vi "Stop Shooter.vi"   [LabVIEW 2013]
uses:
  Shooter Manual Control.ctl
  Shooter Command.ctl
  Robot Global Data.vi
types:
  T1 = typedef "Shooter Manual Control.ctl" = cluster{"Command":T2, "Offset":dbl, "Trigger":bool, "Add":bool, "Release":bool, "Reset":bool, "Target Pressure":dbl, "Punch":bool, "AutoPunch":bool}
  T2 = typedef "Shooter Command.ctl" = enum16{"None", "Warmup", "Shoot", "Line Shoot", "Soft Shoot", "Toss"}
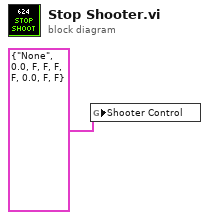
[diagram p0: block diagram]
diagram:
  n1 = global write "Robot Global Data.vi" "Shooter Control"(T1 {"Command"=enum."None", "Offset"=0.0, "Trigger"=FALSE, "Add"=FALSE, "Release"=FALSE, "Reset"=FALSE, "Target Pressure"=0.0, "Punch"=FALSE, "AutoPunch"=FALSE} ("Shooter Control")) -> ()
